vi "Check Engine Blocks Order.vi"(8 "error in (no error)":errorcluster, 10 "previous channel block":T1 {"string descriptor"."buffer offset" format="%d bytes"; "engine descriptor"."buffer offset" format="%d bytes"}, 11 "channel block":T1 {"string descriptor"."buffer offset" format="%d bytes"; "engine descriptor"."buffer offset" format="%d bytes"}) -> (0 "error out":errorcluster)   [LabVIEW 2017, in "DSF Core.lvlib"]
uses:
  DSF Core.lvlib
  Controls/DSF Engine Channel Configuration.ctl
  Controls/DSF Channel Buffer Descriptor.ctl
  Controls/DSF Data Type.ctl
  Channel Overlap.vi
  Shared/VIs/Sizeof.vi
  New Configuration Error.vi
  <vilib>/NI/Memory Manager/VIs/Source.Write.String.vi
  <vilib>/NI/Memory Manager/VIs/Source.Write.Scalar.Base10.vi
  <vilib>/NI/Memory Manager/VIs/Source.Write.Scalar.Base10 (U64).vi
  Shared/Constants/Constants.vi
  Shared/Constants/Engine Library Name.vi
  <vilib>/NI/Memory Manager/VIs/Error Cluster.Set VI Source.vi
  <vilib>/NI/Memory Manager/VIs/Error Cluster.Set Code.vi
  <vilib>/NI/Memory Manager/VIs/Error Cluster.Set Status.vi
  <vilib>/NI/Memory Manager/VIs/New Error Cluster Constant.vi
  <vilib>/NI/Memory Manager/VIs/New Error Cluster Constant (512B).vi
  Configuration Error Info.vi
  Shared/Constants/Base Error Code.vi
  Shared/Constants/Error Offset (Configuration).vi
  Configuration Session.lvclass
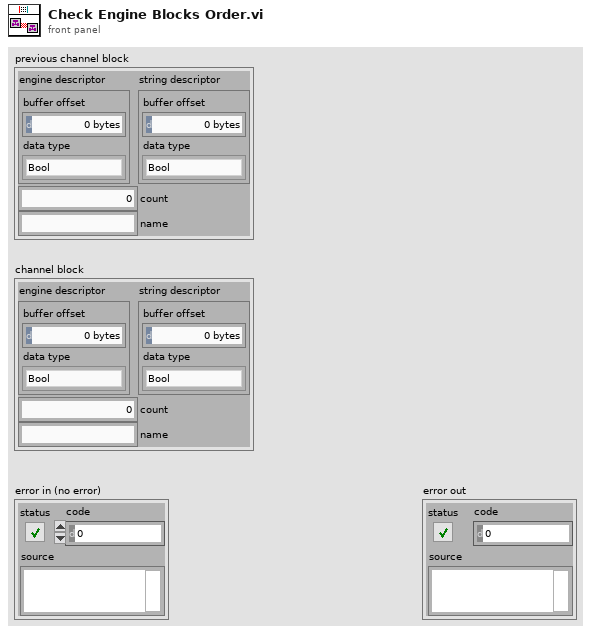
[diagram p1: front panel]
types:
  T1 = typedef "DSF Core.lvlib/DSF Engine Channel Configuration.ctl" = cluster{"engine descriptor":T2, "string descriptor":T2, "count":u64, "name":string}
  T2 = typedef "DSF Core.lvlib/DSF Channel Buffer Descriptor.ctl" = cluster{"buffer offset":u64, "data type":T3}
  T3 = typedef "DSF Core.lvlib/DSF Data Type.ctl" = enum8{"Bool", "SGL", "DBL", "I8", "I16", "I32", "I64", "U8", "U16", "U32", "U64"}
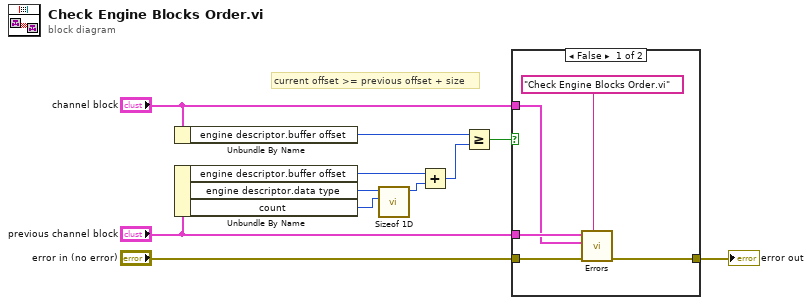
[diagram p0: block diagram]
diagram:
  # "current offset >= previous offset + size"
  n1 = Unbundle By Name("channel block") -> ("engine descriptor.buffer offset"=w4:u64)
  n2 = Unbundle By Name("previous channel block") -> ("engine descriptor.buffer offset"=w7:u64, "engine descriptor.data type"=w6:T3, "count"=w1:u64)
  n3 = call "Sizeof 1D.vi"("count"=w1, "data type"=w6) -> ("size in bytes"=w8:u64)  [unwired: 9 in]
  n4 = Add(x=w7, y=w8) -> (x+y=w3:u64)
  n5 = Greater Or Equal?(x=w4, y=w3) -> (x >= y?=w2:bool)
  n6 = case shown="False" w2 {
    tunnel: "previous channel block" -> [w16 _]
    tunnel: "channel block" -> [w15 _]
    tunnel: [w14 w17] -> w10
    tunnel: "error in (no error)" -> [w13 w17]
    frame False {
      n7 = call-poly "Errors.vi"("error source vi name"="Check Engine Blocks Order.vi", "error in (no error)"=w13, "current channel block"=w15, "previous channel block"=w16) -> ("error out"=w14:errorcluster)  [unwired: 7 in]
    }
    frame True {
      # "Valid. Proceed."
    }
  }
  "error out" <- w10
